vi "Configure Channel Trigger.vi"(7 "Units (0: Volt)":i32(ring) items=["Volt", "Ampere"], 8 "error in (no error)":errorcluster, 9 "Vertical Range (8.0 V)":dbl=8.0, 10 "Probe Attenuation Factor (1.0 X)":dbl=1.0, 11 "VISA resource name":refnum<visa-resource-name>) -> (0 "error out":errorcluster, 3 "VISA resource name out":refnum<visa-resource-name>)   [LabVIEW 2015, in "Agilent 2000 3000 X-Series.lvlib"]
doc: "Configures the channel setting for External Trigger."
uses:
  <instrlib>/Agilent 2000 3000 X-Series/Agilent 2000 3000 X-Series.lvlib
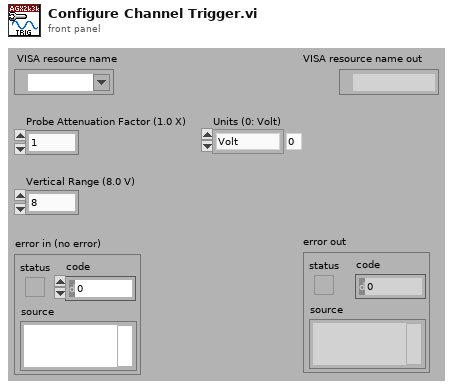
[diagram p1: front panel]
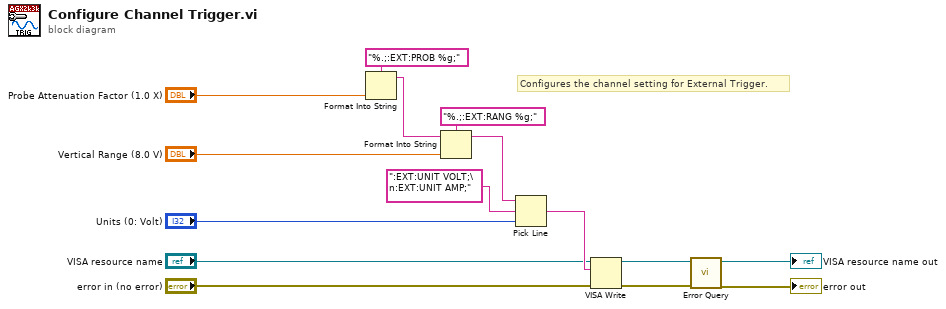
[diagram p0: block diagram]
diagram:
  # "Configures the channel setting for External Trigger."
  n1 = Format Into String(format string="%.;:EXT:PROB %g;", "Probe Attenuation Factor (1.0 X)") -> (resulting string=w13:string)  [unwired: 2 in, 1 out]
  n2 = Format Into String(format string="%.;:EXT:RANG %g;", initial string=w13, "Vertical Range (8.0 V)") -> (resulting string=w8:string)  [unwired: 1 in, 1 out]
  n3 = Pick Line(string ("")=w8, multi-line string=":EXT:UNIT VOLT;\n:EXT:UNIT AMP;", line index="Units (0: Volt)") -> (output string=w7:string)
  n4 = VISA Write(VISA resource name="VISA resource name", write buffer=w7, error in (no error)="error in (no error)") -> (VISA resource name out=w4:refnum<visa-resource-name>, error out=w3:errorcluster)  [unwired: 1 out]
  n5 = call <instrlib>:"Error Query.vi"("error in (no error)"=w3, "VISA resource name"=w4) -> ("error out"=→"error out":errorcluster, "VISA resource name out"=→"VISA resource name out":refnum<visa-resource-name>)  [unwired: 8 out]
